vi "Query-Melt-characteristics-needed.vi"(8 "error in":errorcluster, 10 "Correct. params. ref.":refnum<data-value>, 11 "Temp. params. ref.":refnum<data-value>) -> (0 "error IO":errorcluster, 3 "Melt characteristics?":bool)   [LabVIEW 2013, in "CameraVision.lvlib" / "CV-Analysis.lvclass"]
uses:
  CV-Analysis.lvclass
  Temperature/CV-Temperature.lvclass
  Correction/CV-Correction.lvclass
  Correction/CV-Correction.lvclass/CV-Correction.ctl
  Temperature/CV-Temperature.lvclass/CV-Temperature.ctl
  Temperature/Read Temperature field.vi
  Temperature/Read Temperature value.vi
  Temperature/Read Averaging shape.vi
  Temperature/Read Averaging center.vi
  Correction/Read Correlation algorithm.vi
  Correction/Read 2nd image correlation.vi
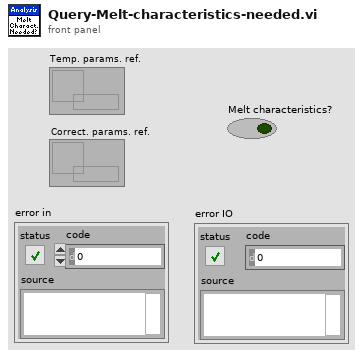
[diagram p1: front panel]
types:
  T1 = enum16{"Fixed shift", "Cross-correlation", "Cross-correlation (5steps)", "Melt-pool center"}
  T2 = enum16{"Fixed coordinates (pixel)", "Fixed coordinates (mm)", "Melt-pool center"}
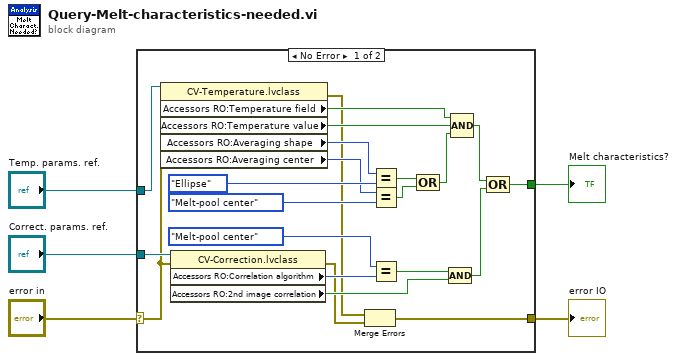
[diagram p0: block diagram]
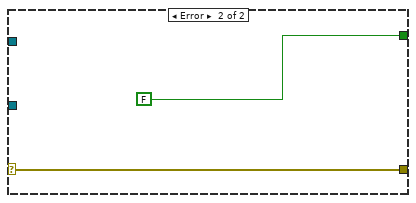
[diagram p2: hidden frame]
diagram:
  n1 = case shown="No Error" "error in" {
    selector: "error in" -> [w9 w28]
    tunnel: [w23 FALSE] -> w5
    tunnel: "Temp. params. ref." -> [w17 _]
    tunnel: [w8 w28] -> w3
    tunnel: "Correct. params. ref." -> [w12 _]
    frame No Error {
      n2 = property class="CV-Temperature.lvclass"(reference=w17, error in=w9) -> (error out=w7:errorcluster, "Accessors RO:Temperature field"=w16:bool, "Accessors RO:Temperature value"=w15:bool, "Accessors RO:Averaging shape"=w14:enum16{"Point", "Circle", "Ellipse"}, "Accessors RO:Averaging center"=w13:T2)  [unwired: 1 out]
      n3 = property class="CV-Correction.lvclass"(reference=w12, error in=w9) -> (error out=w6:errorcluster, "Accessors RO:Correlation algorithm"=w11:T1, "Accessors RO:2nd image correlation"=w10:bool)  [unwired: 1 out]
      n4 = Merge Errors(w7, w6) -> (w8:errorcluster)
      n5 = Equal?(x=w14, y=enum16{"Point", "Circle", "Ellipse"}."Ellipse" ("x")) -> (x = y?=w26:bool)
      n6 = Equal?(x=w13, y=T2."Melt-pool center" ("x")) -> (x = y?=w27:bool)
      n7 = Equal?(x=T1."Melt-pool center" ("y"), y=w11) -> (x = y?=w20:bool)
      n8 = Compound Arithmetic op=OR(w26, w27) -> (w18:bool)
      n9 = Compound Arithmetic op=AND(w20, w10) -> (w19:bool)
      n10 = Compound Arithmetic op=AND(w16, w15, w18) -> (w22:bool)
      n11 = Compound Arithmetic op=OR(w22, w19) -> (w23:bool)
    }
    frame Error {
    }
  }
  "Melt characteristics?" <- w5
  "error IO" <- w3
